vi "DetectorReadData-2D.vi"(0 "Microscope in":refnum<class "Microscope.lvclass">, 1 "Detector Type":T1, 3 "Actual Samples Per Line":i32, 4 "Computed Parameter.Samples to Average":i32, 5 "Computed Parameter.Trash Samples":i32, 7 "Digital Image Multiplier":dbl[](array[numeric]), 8 "Threshold":dbl[](array[numeric])=[0.0, 0.0, 0.0], 9 "error in (no error)":errorcluster, 10 "Threshold defaults":dbl[](array[numeric])=[0.0, 0.0, 0.0], 11 "show flyback data":bool, 13 "disable averaging":bool) -> (14 "Microscope out":refnum<class "Microscope.lvclass">, 15 "Data":dbl[][](array[numeric]), 19 "error out":errorcluster)   [LabVIEW 2012, in "Microscope.lvclass"]
uses:
  classes/Microscope.lvclass
  typedefs/DetectorType.ctl
  classes/Microscope.lvclass/Microscope.ctl
  <vilib>/DAQmx/read.llb/DAQmx Read (Analog 2D DBL NChan NSamp).vi
  <vilib>/DAQmx/miscellaneous.llb/DAQmx Fill In Error Info.vi
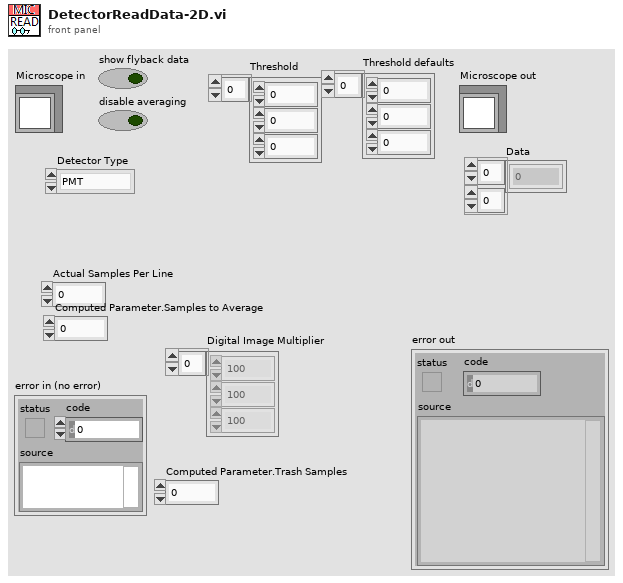
[diagram p1: front panel]
types:
  T1 = typedef "DetectorType.ctl" = enum16{"PMT", "SpectraWiz"}
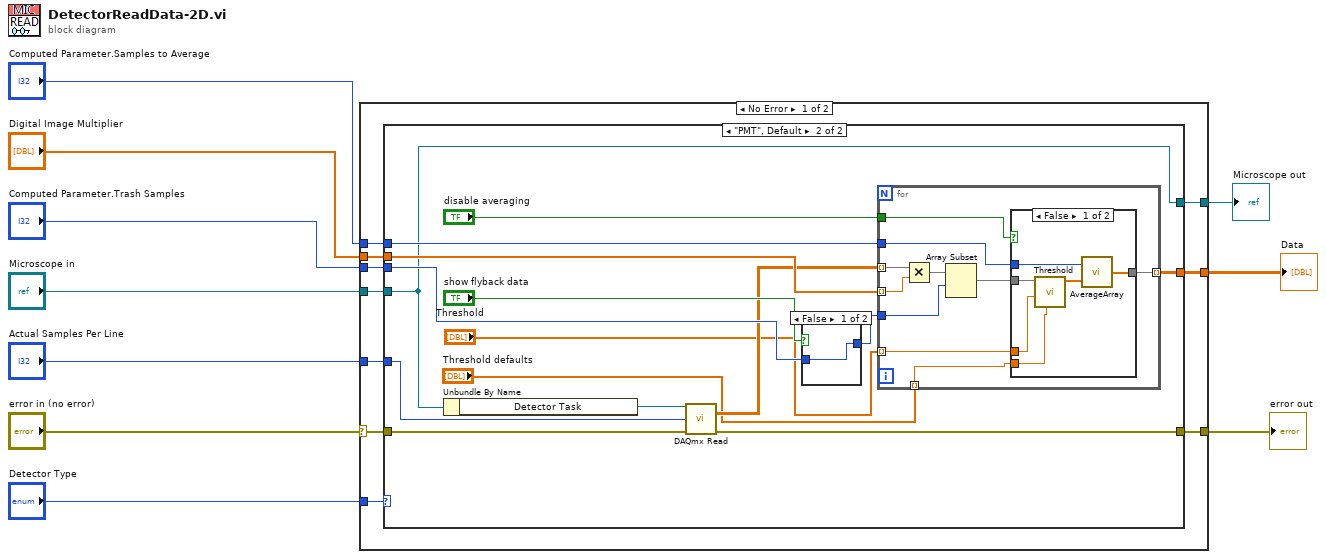
[diagram p0: block diagram]
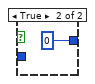
[diagram p3: hidden frame]
diagram:
  n1 = case shown="No Error" "error in (no error)" {
    selector: "error in (no error)" -> [w19 w58]
    tunnel: [w17 w58] -> w9
    tunnel: [w18 w57] -> w7
    tunnel: "Microscope in" -> [w16 w57]
    tunnel: [w20 _] -> w6
    tunnel: "Detector Type" -> [w15 _]
    tunnel: "Digital Image Multiplier" -> [w14 _]
    tunnel: "Actual Samples Per Line" -> [w13 _]
    tunnel: "Computed Parameter.Samples to Average" -> [w12 _]
    tunnel: "Computed Parameter.Trash Samples" -> [w11 _]
    frame No Error {
      n2 = case shown="\"PMT\", Default" w15 {
        tunnel: [_ w37] -> w20
        tunnel: w19 -> [w21 w36]
        tunnel: [w22 w24] -> w18
        tunnel: [w21 w35] -> w17
        tunnel: w16 -> [w22 w24]
        tunnel: w14 -> [_ w34]
        tunnel: w13 -> [_ w33]
        tunnel: w12 -> [_ w32]
        tunnel: w11 -> [_ w31]
        frame "SpectraWiz" {
        }
        frame "PMT", Default {
          n3 = Unbundle By Name(w24) -> ("Detector Task"=w30:refnum<k21>)
          n4 = call-poly <vilib>:"DAQmx Read.vi"("task/channels in"=w30, "number of samples per channel"=w33, "error in"=w36) -> ("data"=w26:dbl[][], "error out"=w35:errorcluster)  [unwired: 10 in, 1 out]
          n5 = case shown="False" "show flyback data" {
            tunnel: w31 -> [w38 _]
            tunnel: [w38 0 ("Trash Samples")] -> w27
            frame False {
            }
            frame True {
            }
          }
          n6 = for {
            tunnel: w32 -> [w49]
            tunnel: "disable averaging" -> [w48]
            tunnel: w27 -> [w47]
            tunnel: [w45] -> w37 mode=indexing
            tunnel: w26 -> [w43] mode=indexing
            tunnel: w34 -> [w42] mode=indexing
            tunnel: "Threshold" -> [w41] mode=indexing
            tunnel: "Threshold defaults" -> [w40] mode=indexing
            n7 = Multiply(x=w43, y=w42) -> (x*y=w44:dbl[])
            n8 = Array Subset(array=w44, index=w47) -> (w46:dbl[])  [unwired: 1 in]
            n9 = case shown="False" w48 {
              tunnel: w46 -> [w53 w56]
              tunnel: w49 -> [w55 _]
              tunnel: [w54 w56] -> w45
              tunnel: w41 -> [w51 _]
              tunnel: w40 -> [w50 _]
              frame False {
                n10 = call "Threshold.vi"("Default value"=w50, "Threshold value"=w51, "Input data values"=w53) -> ("Thresholded data values"=w52:dbl[])  [unwired: 8 in]
                n11 = call "AverageArray.vi"("Input Array"=w52, "Samples To Average"=w55) -> ("Averaged Array"=w54:dbl[])
              }
              frame True {
              }
            }
          }
        }
      }
    }
    frame Error {
    }
  }
  "error out" <- w9
  "Microscope out" <- w7
  "Data" <- w6
